vi "Teleop.vi"(10 "Match Info":T1={"Autonomous Elapsed Seconds"=0.0, "TeleOp Elapsed Seconds"=0.0, "Disabled Elapsed Seconds"=0.0, "Visited Autonomous"=FALSE, "Visited TeleOp"=FALSE, "Visited Disabled"=FALSE, "Autonomous Settings"={"Autonomous Style"=enum."Independent", "VI Refnum"=refnum}}, 11 "Call Context":T2) -> ()   [LabVIEW 2015]
doc: "This VI is called for each TeleOp packet received from the DS where the robot is not disabled. It is often used to read from the joysticks and update I/O or to update setpoints for timed control loops. It should complete and return within 20 milliseconds or it may miss DS packets."
uses:
  <vilib>/Rock Robotics/WPI/DriverStation/WPI_DriverStationDerivedRobotMode.ctl
  <vilib>/Rock Robotics/WPI/DriverStation/WPI_DriverStationMatch Info.ctl
  <vilib>/Rock Robotics/Network Tables/NT Read Boolean.vi
  <vilib>/Rock Robotics/Network Tables/NT Read Number.vi
  Team900-VIs/Logitech/F510/F510-X.vi
  <vilib>/Rock Robotics/Network Tables/NT Write Numeric Array.vi
  Robot Global Data.vi
  Team900-VIs/Team900SwerveDrive/Team900SwerveDrive.lvlib
  Team900-VIs/navX Library v2/navX Library v2.lvlib
panel:
  in  "Force Aim":bool=TRUE
  out "Waveform Chart":cluster{dbl, dbl, dbl, dbl}(graph)
  in  "Negate?":bool=TRUE
  in  "Max Wheel Speed (Ticks per tenth of a second?)":dbl=20000.0
  out "Sample Slider 0":dbl(slide) scale=0.0..5.0
  out "Sample Boolean 1":bool
  out "Sample Boolean 0":bool
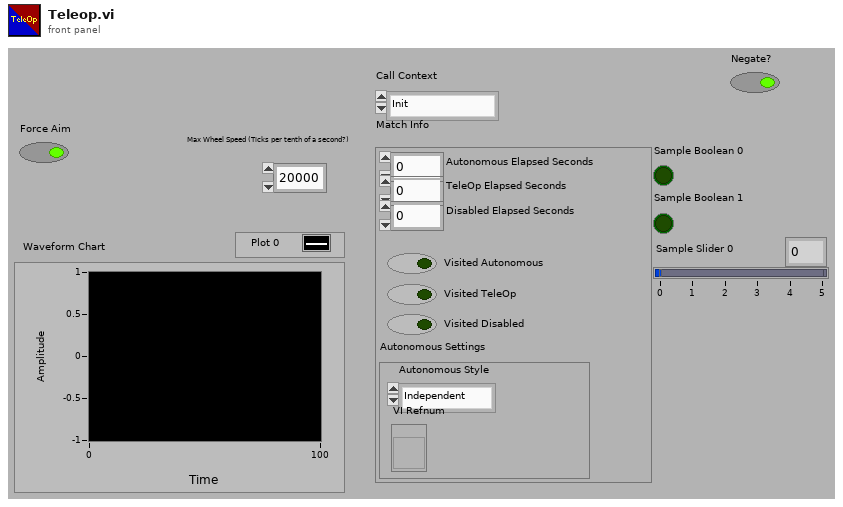
[diagram p1: front panel]
types:
  T1 = typedef "WPI_DriverStationMatch Info.ctl" = cluster{"Autonomous Elapsed Seconds":dbl, "TeleOp Elapsed Seconds":dbl, "Disabled Elapsed Seconds":dbl, "Visited Autonomous":bool, "Visited TeleOp":bool, "Visited Disabled":bool, "Autonomous Settings":cluster{"Autonomous Style":enum16{"Iterative", "Independent"}, "VI Refnum":refnum<vi>}}
  T2 = typedef "WPI_DriverStationDerivedRobotMode.ctl" = enum16{"Init", "Execute", "Stop"}
  T3 = enum16{"nothing", "Fire", "Aim Goal", "Aim Foward"}
  T4 = enum16{"nothing", "intaketotop", "eject ball", "load ball to shooter", "intaketobottom"}
  T5 = cluster{"A":bool, "B":bool, "X":bool, "Y":bool, "LB":bool, "RB":bool, "Back":bool, "Start":bool, "LC":bool, "RC":bool, "LT":bool, "RT":bool}
  T6 = cluster{"Up":bool, "Right":bool, "Down":bool, "Left":bool}
  T7 = typedef "navX Library v2.lvlib/Z900_navX_DeviceTypeDef.ctl" = cluster{"Interface":cluster{"Protocol":T8, "Update Rate (4Hz-60Hz)":u8, "navX Open TypeDef":variant}, "Notify Packet":refnum<notifier>, "Loop VI Refnum":refnum<vi>, "Ready to Close Occurrence Refnum":refnum<k4>}
  T8 = typedef "navX Library v2.lvlib/Z900_navX_ProtocolTypeDef.ctl" = enum16{"SERIAL", "I2C", "SPI"}
  T9 = cluster{"Yaw":dbl, "Roll":dbl, "Pitch":dbl, "Heading":dbl, "Fused Heading":dbl}
  T10 = typedef "WPI_MotorControlDeviceRef.ctl" = cluster{"DeviceStatus":errorcluster, "Type":T11, "PWM":cluster{"PWM Channel":T12, "DeadBand":T13}, "CAN":cluster{"Device Number":u8, "Control Mode":T14, "Semaphore":T15, "Max Vout":dbl, "TalonSRX Control Mode":T16}, "Invert":bool}
  T11 = typedef "WPI_MotorControlType.ctl" = enum16{"PWM", "CAN", "CANTalonSRX"}
  T12 = typedef "FPGA_DIOPWMChannel.ctl" = enum8{"PWM 0", "PWM 1", "PWM 2", "PWM 3", "PWM 4", "PWM 5", "PWM 6", "PWM 7", "PWM 8", "PWM 9", "PWM MXP 0", "PWM MXP 1", "PWM MXP 2", "PWM MXP 3", "PWM MXP 4", "PWM MXP 5", "PWM MXP 6", "PWM MXP 7", "PWM MXP 8", "PWM MXP 9", "Invalid"}
  T13 = typedef "WPI_PWMDeadband.ctl" = cluster{"Name":string, "maxPositivePwm":i32, "minPositivePwm":i32, "centerPwm":i32, "maxNegativePwm":i32, "minNegativePwm":i32, "angularRange":u16}
  T14 = typedef "WPI_CANJaguar_ControlMode.ctl" = enum8{"Percent VBus", "Current", "Speed", "Position", "Voltage"}
  T15 = typedef "Semaphore RefNum" = refnum<k1>
  T16 = typedef "WPI_CANTalonSRX_APIControlMode.ctl" = enum8{"Percent VBus", "Speed", "Position", "Slave", "Unchanged / Invalid", "Voltage Compensation", "Current", "Motion Profile"}
  T17 = typedef "WPI_CANTalonSRX_GlobalStatus.ctl" = cluster{"Applied Throttle":dbl, "Module Enabled":bool, "CAN Error":errorcluster, "Closed Loop Error":dbl, "Forward Limit Switch Closed":bool, "Reverse Limit Switch Closed":bool, "Sensor Position":dbl, "Sensor Velocity":dbl, "Current":dbl, "Sticky Fault - Over Temp":bool, "Sticky Fault - Under Voltage":bool, "Sticky Fault - Forward Limit":bool, "Sticky Fault - Reverse Limit":bool, "Sticky Fault - Forward Soft Limit":bool, "Sticky Fault - Reverse Soft Limit":bool, "Brake is Enabled":bool, "Encoder Position":dbl, "Encoder Velocity":dbl, "Encoder Index Count":dbl, "Encoder A Pin State":bool, "Encoder B Pin State":bool, "Encoder Index Pin State":bool, "Analog In":dbl, "Analog In Velocity":dbl, "Temperature (C)":dbl, "Battery Voltage":dbl, "Control 5 Is Supported":bool, "Current Profile Slot Select":dbl, "Pos Div 8":bool, "Vel Div 4":bool, "Pulse Width Position":i32, "Pulse Width Velocity":i32, "Pulse Width Rise To Rise (us)":i32, "Pulse Width Rise To Fall (us)":i32, "Mot Prof Active Is Under Run":bool, "Mot Prof Active Has Under Run":bool, "Mot Prof Active Is Last":bool, "Mot Prof Active Velocity Only":bool, "Mot Prof Active Is Valid":bool, "Mot Prof Buffer Is Full":bool, "Mot Prof Active Profile Slot Select":i32, "Mot Prof NextID":i32, "Mot Prof Count":i32, "Mot Prof Active Velocity":dbl, "Mot Prof Active Position":dbl, "Mot Prof Output Enable":i32}
  T18 = typedef "WPI_DigitalInputDevRef.ctl" = cluster{"DevStatus":errorcluster, "DIO Channel":T19}
  T19 = typedef "FPGA_DIOChannel.ctl" = enum8{"DIO 0", "DIO 1", "DIO 2", "DIO 3", "DIO 4", "DIO 5", "DIO 6", "DIO 7", "DIO 8", "DIO 9", "DIO MXP 0", "DIO MXP 1", "DIO MXP 2", "DIO MXP 3", "DIO MXP 4", "DIO MXP 5", "DIO MXP 6", "DIO MXP 7", "DIO MXP 8", "DIO MXP 9", "DIO MXP 10", "DIO MXP 11", "DIO MXP 12", "DIO MXP 13", "DIO MXP 14", "DIO MXP 15", "Invalid"}
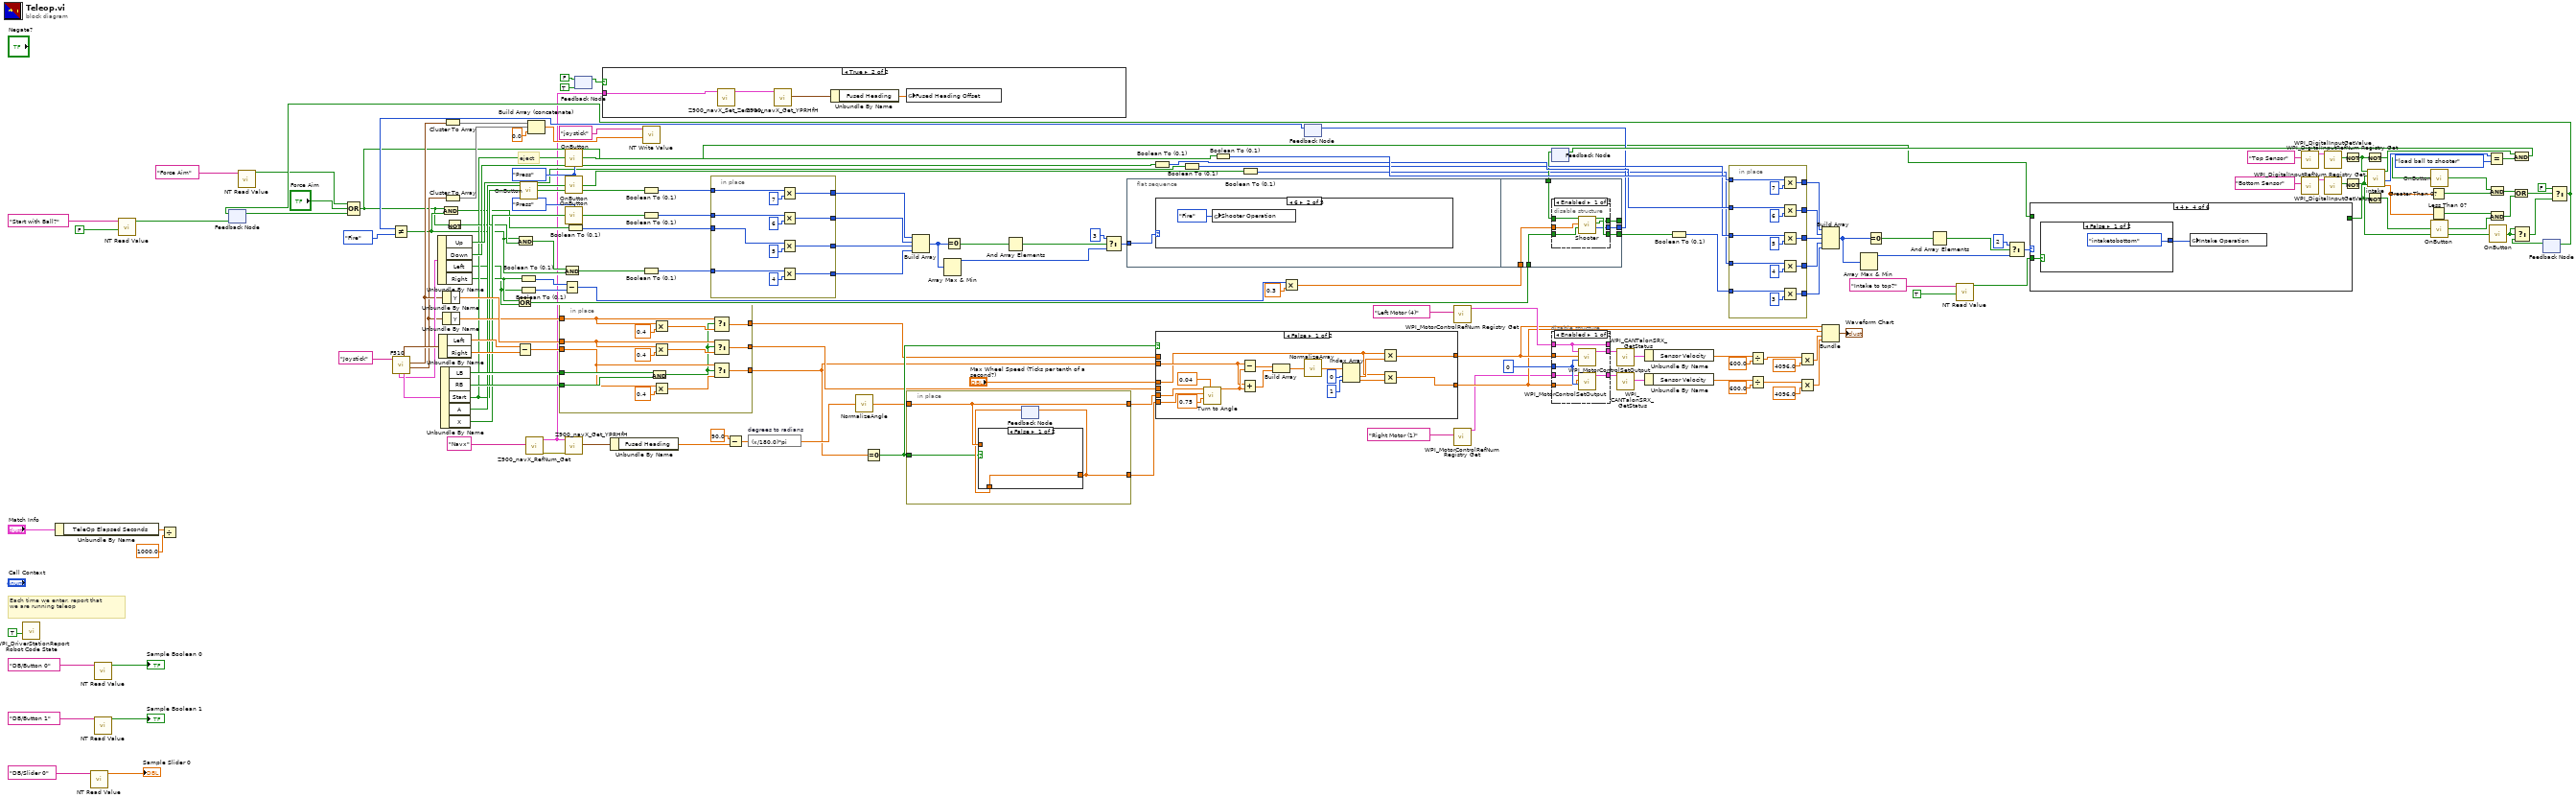
[diagram p0: block diagram]
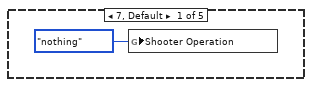
[diagram p4: hidden frame]
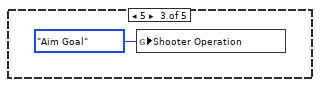
[diagram p5: hidden frame]
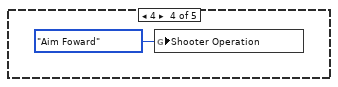
[diagram p6: hidden frame]
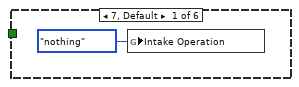
[diagram p9: hidden frame]
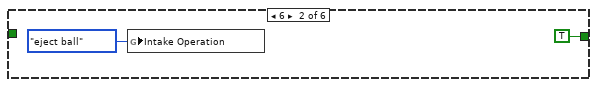
[diagram p10: hidden frame]
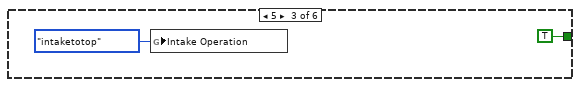
[diagram p11: hidden frame]
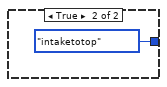
[diagram p12: hidden frame]
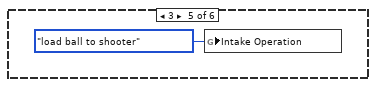
[diagram p13: hidden frame]
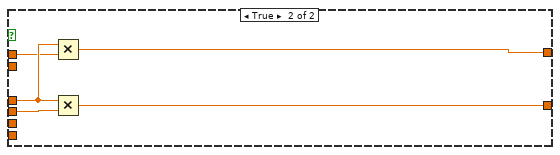
[diagram p16: hidden frame]
diagram:
  w130 = enum16{"Press", "Release", "Both"}."Press" ("Mode")
  # "eject"
  # "Each time we enter, report that\nwe are running teleop"
  n1 = call <vilib>:"WPI_DriverStationReport Robot Code State.vi"("TeleOp"=TRUE ("Autonomous")) -> ()  [unwired: 10 in, 1 out]
  n2 = Unbundle By Name("Match Info") -> ("TeleOp Elapsed Seconds"=w134:dbl)
  n3 = call-poly <vilib>:"NT Read Value.vi"("Name"="DB/Slider 0" ("refnum name")) -> ("Numeric"=→"Sample Slider 0":dbl)  [unwired: 9 in, 1 out]
  n4 = call-poly <vilib>:"NT Read Value.vi"("Name"="DB/Button 0" ("refnum name")) -> ("Boolean"=→"Sample Boolean 0":bool)  [unwired: 9 in, 1 out]
  n5 = call-poly <vilib>:"NT Read Value.vi"("Name"="DB/Button 1" ("refnum name")) -> ("Boolean"=→"Sample Boolean 1":bool)  [unwired: 9 in, 1 out]
  n6 = call-poly <vilib>:"NT Read Value.vi"("Default Value"=FALSE, "Name"="Start with Ball?") -> ("Boolean"=w17:bool)  [unwired: 8 in, 1 out]
  n7 = Divide(x=w134, y=1000.0) -> ()  [unwired: 1 out]
  n8 = feedback #1(w17) -> (w25:bool)
  n9 = call-poly <vilib>:"NT Read Value.vi"("Name"="Force Aim") -> ("Boolean"=w15:bool)  [unwired: 9 in, 1 out]
  n10 = Compound Arithmetic op=OR(w15, "Force Aim", w25) -> (w40:bool)
  n11 = call-poly "F510.vi"("refnum name"="Joystick") -> ("Right Stick"=w74:cluster{"X":dbl, "Y":dbl}, "Left Stick"=w75:cluster{"X":dbl, "Y":dbl}, "Buttons"=w155:T5, "Triggers"=w154:cluster{"Left":dbl, "Right":dbl}, "D-Pad Buttons"=w132:T6)  [unwired: 4 in, 2 out]
  n12 = Unbundle By Name(w132) -> ("Up"=w104:bool, "Down"=w103:bool, "Left"=w6:bool, "Right"=w7:bool)
  n13 = Unbundle By Name(w154) -> ("Left"=w153:dbl, "Right"=w152:dbl)
  n14 = Unbundle By Name(w155) -> ("LB"=w159:bool, "RB"=w160:bool, "Start"=w85:bool, "A"=w131:bool, "X"=w102:bool)
  n15 = Unbundle By Name(w75) -> ("Y"=w157:dbl)
  n16 = Unbundle By Name(w74) -> ("Y"=w158:dbl)
  n17 = Cluster To Array(cluster=w75) -> (array=w73:dbl[])
  n18 = Cluster To Array(cluster=w74) -> (array=w72:dbl[])
  n19 = Not(x=w40) -> (.not. x?=w88:bool)
  n20 = Or(x=w7, y=w6) -> (x .or. y?=w5:bool)
  n21 = Subtract(x=w153, y=w152) -> (x-y=w112:dbl)
  n22 = Boolean To (0,1)(Boolean=w7) -> (0, 1=w12:i16)
  n23 = Boolean To (0,1)(Boolean=w6) -> (0, 1=w11:i16)
  n24 = call "OnButton.vi"("Button"=w85) -> ("Value"=w86:bool)  [unwired: 1 in]
  n25 = call "Z900_navX_RefNum_Get.vi"("refnum name"="Navx") -> ("error out"=w139:errorcluster, "navX Device"=w1:T7)  [unwired: 9 in]
  n26 = Build Array (concatenate)(w73, w72, 0.0) -> (w69:dbl[])
  n27 = in-place {
    in-place-border: w160 -> [w183]
    in-place-border: w159 -> [w182]
    in-place-border: w158 -> [w177]
    in-place-border: w157 -> [w176]
    in-place-border: [w175] -> w79
    in-place-border: [w174] -> w145
    in-place-border: w112 -> [w171]
    in-place-border: [w169] -> w111
    n28 = And(x=w182, y=w183) -> (x .and. y?=w170:bool)
    n29 = Multiply(x=w176, y=0.4) -> (x*y=w179:dbl)
    n30 = Multiply(x=w177, y=0.4) -> (x*y=w181:dbl)
    n31 = Multiply(x=w171, y=0.4) -> (x*y=w173:dbl)
    n32 = Select(t=w176, s=w170, f=w179) -> (s? t:f=w175:dbl)
    n33 = Select(t=w177, s=w170, f=w181) -> (s? t:f=w174:dbl)
    n34 = Select(t=w171, s=w170, f=w173) -> (s? t:f=w169:dbl)
  }
  n35 = Subtract(x=w12, y=w11) -> (x-y=w9:i16)
  n36 = call "OnButton.vi"("Button"=w85, "Mode"=w130) -> ("Value"=w47:bool)
  n37 = call "OnButton.vi"("Button"=w131, "Mode"=w130) -> ("Value"=w43:bool)
  n38 = call "OnButton.vi"("Button"=w102, "Mode"=enum16{"Press", "Release", "Both"}."Press") -> ("Value"=w100:bool)
  n39 = call "Z900_navX_Get_YPRHfH.vi"("error in (no error)"=w139, "navX Device"=w1) -> ("YRPHfH"=w140:T9)  [unwired: 6 in, 3 out]
  n40 = feedback-in #2(FALSE) -> ()
  n41 = feedback #2(TRUE) -> (w3:bool)
  n42 = case shown="True" w3 {
    tunnel: w1 -> [_ w184]
    frame False {
    }
    frame True {
      n43 = call "Z900_navX_Set_ZeroYaw.vi"("navX Device"=w184) -> ("navX Device"=w185:T7)  [unwired: 9 in, 1 out]
      n44 = call "Z900_navX_Get_YPRHfH.vi"("navX Device"=w185) -> ("YRPHfH"=w187:T9)  [unwired: 7 in, 3 out]
      n45 = Unbundle By Name(w187) -> ("Fused Heading"=w186:dbl)
      n46 = global write "Robot Global Data.vi" "Fused Heading Offset"(w186) -> ()
    }
  }
  n47 = Unbundle By Name(w140) -> ("Fused Heading"=w81:dbl)
  n48 = Boolean To (0,1)(Boolean=w86) -> (0, 1=w83:i16)
  n49 = Boolean To (0,1)(Boolean=w100) -> (0, 1=w99:i16)
  n50 = call-poly <vilib>:"NT Write Value.vi"("Numeric Array"=w69, "Name"="joystick") -> ()  [unwired: 9 in, 1 out]
  n51 = Subtract(x=90.0 ("y"), y=w81) -> (x-y=w136:dbl)
  n52 = expression code="(x/180.0)*pi" "degrees to radians"(w136) -> (w143:dbl)
  n53 = call "NormalizeAngle.vi"("angle (rad)"=w143) -> ("angle (between pi and -pi)"=w142:dbl)
  n54 = Equal To 0?(x=w111) -> (x = 0?=w146:bool)
  n55 = in-place {
    in-place-border: w142 -> [w191]
    in-place-border: w146 -> [w188]
    in-place-border: [w191] -> w144
    in-place-border: [w189] -> w141
    n56 = feedback #3() -> (w190:dbl)  [unwired: 1 in]
    n57 = case shown="False" w188 {
      tunnel: w191 -> [_ w193]
      tunnel: [w192 w193] -> w189
      tunnel: w190 -> [w192 _]
      frame False {
      }
      frame True {
      }
    }
    n58 = feedback-in #3(w189) -> ()
  }
  n59 = flat-sequence {
    tunnel: w87 -> [w194]
    tunnel: w82 -> [w204]
    tunnel: [w203] -> _
    tunnel: [w202] -> w48
    tunnel: [w201] -> w80
    tunnel: w8 -> [w200]
    tunnel: w5 -> [w199]
    frame #0 {
      n60 = case shown="6" w194 {
        frame 7, Default {
          n61 = global write "Robot Global Data.vi" "Shooter Operation"(T3."nothing" ("Shooter Operation")) -> ()
        }
        frame 6 {
          n62 = global write "Robot Global Data.vi" "Shooter Operation"(T3."Fire" ("y")) -> ()
        }
        frame 5 {
          n63 = global write "Robot Global Data.vi" "Shooter Operation"(T3."Aim Goal" ("Shooter Operation")) -> ()
        }
        frame 4 {
          n64 = global write "Robot Global Data.vi" "Shooter Operation"(T3."Aim Foward" ("Shooter Operation")) -> ()
        }
        frame 3 {
        }
      }
    }
    frame #1 {
      n65 = disable-structure shown="Enabled" {
        disable-tunnel: [w210 _] -> w202
        disable-tunnel: w204 -> [w209 _]
        disable-tunnel: [w208 _] -> w201
        disable-tunnel: [w207 _] -> w203
        disable-tunnel: w200 -> [w206 _]
        disable-tunnel: w199 -> [w205 _]
        frame Enabled {
          n66 = call "Shooter.vi"("Override?"=w205, "Override Setpoint"=w206, "Load Ball Finished"=w209) -> ("Shooter Operation"=w208:T3, "Finished"=w207:bool, "Load Ball"=w210:bool)  [unwired: 5 in, 1 out]
        }
        frame Disabled {
        }
      }
    }
  }
  n67 = Boolean To (0,1)(Boolean=w103) -> (0, 1=w128:i16)
  n68 = case shown="False" w146 {
    tunnel: "Max Wheel Speed (Ticks per tenth of a second?)" -> [w213 w230]
    tunnel: [w225 w231] -> w67
    tunnel: [w226 w232] -> w68
    tunnel: w144 -> [w211 _]
    tunnel: w111 -> [w222 _]
    tunnel: w79 -> [_ w229]
    tunnel: w145 -> [_ w228]
    tunnel: w141 -> [w212 _]
    frame False {
      n69 = call "Turn to Angle.vi"("Angle Tolerance"=0.04, "Rotation Multiplier"=0.75, "Target angle"=w212, "Angle (radians; 0 = right)"=w211) -> ("Turn Set Point"=w223:dbl)  [unwired: 3 in, 1 out]
      n70 = Subtract(x=w222, y=w223) -> (x-y=w221:dbl)
      n71 = Add(x=w222, y=w223) -> (x+y=w214:dbl)
      n72 = Build Array(w221, w214) -> (w220:dbl[])
      n73 = call "NormalizeArray.vi"("array"=w220) -> ("normalized array"=w219:dbl[])
      n74 = Index Array(array=w219, index #1=0 ("index"), index #2=1 ("index")) -> (element #1=w216:dbl, element #2=w215:dbl)
      n75 = Multiply(x=w213, y=w216) -> (x*y=w226:dbl)
      n76 = Multiply(x=w213, y=w215) -> (x*y=w225:dbl)
    }
    frame True {
      n77 = Multiply(x=w230, y=w229) -> (x*y=w232:dbl)
      n78 = Multiply(x=w230, y=w228) -> (x*y=w231:dbl)
    }
  }
  n79 = Boolean To (0,1)(Boolean=w104) -> (0, 1=w127:i16)
  n80 = Boolean To (0,1)(Boolean=w47) -> (0, 1=w129:i16)
  n81 = Boolean To (0,1)(Boolean=w43) -> (0, 1=w46:i16)
  n82 = Multiply(x=w9, y=0.3) -> (x*y=w8:dbl)
  n83 = feedback #4() -> (w77:T3)  [unwired: 1 in]
  n84 = Not Equal?(x=w77, y=T3."Fire") -> (x != y?=w49:bool)
  n85 = And(x=w40, y=w49) -> (x .and. y?=w41:bool)
  n86 = And(x=w49, y=w88) -> (x .and. y?=w50:bool)
  n87 = And(x=w50, y=w49) -> (x .and. y?=w78:bool)
  n88 = Boolean To (0,1)(Boolean=w41) -> (0, 1=w90:i16)
  n89 = Boolean To (0,1)(Boolean=w78) -> (0, 1=w89:i16)
  n90 = in-place {
    in-place-border: w99 -> [w244]
    in-place-border: w90 -> [w241]
    in-place-border: w89 -> [w239]
    in-place-border: [w238] -> w93
    in-place-border: [w237] -> w92
    in-place-border: [w236] -> w91
    in-place-border: w83 -> [w234]
    in-place-border: [w233] -> w84
    n91 = Multiply(x=w234, y=i16 7) -> (x*y=w233:i16)
    n92 = Multiply(x=w244, y=i16 6) -> (x*y=w238:i16)
    n93 = Multiply(x=w241, y=i16 5) -> (x*y=w237:i16)
    n94 = Multiply(x=w239, y=i16 4) -> (x*y=w236:i16)
  }
  n95 = Build Array(w84, w93, w92, w91) -> (w98:i16[])
  n96 = Array Max & Min(array=w98) -> (max value=w94:i16)  [unwired: 3 out]
  n97 = Equal To 0?(x=w98) -> (x = 0?=w97:bool[])
  n98 = And Array Elements(Boolean array=w97) -> (logical AND=w96:bool)
  n99 = Select(t=3, s=w96, f=w94) -> (s? t:f=w87:i32)
  n100 = feedback-in #4(w80) -> ()
  n101 = call <vilib>:"WPI_MotorControlRefNum Registry Get.vi"("refnum name"="Left Motor (4)") -> ("MotorControlDevRef"=w148:T10)  [unwired: 9 in, 1 out]
  n102 = call <vilib>:"WPI_MotorControlRefNum Registry Get.vi"("refnum name"="Right Motor (1)") -> ("MotorControlDevRef"=w66:T10)  [unwired: 9 in, 1 out]
  n103 = feedback #5() -> (w82:bool)  [unwired: 1 in]
  n104 = disable-structure shown="Enabled" {
    disable-tunnel: u8 0 ("Sync Group / Parameter Slot") -> [w251 _]
    disable-tunnel: w66 -> [w250 _]
    disable-tunnel: w148 -> [w247 _]
    disable-tunnel: w68 -> [w249 _]
    disable-tunnel: w67 -> [w248 _]
    disable-tunnel: [w247 _] -> _
    disable-tunnel: [w246 _] -> w65
    disable-tunnel: [w245 _] -> w64
    frame Enabled {
      n105 = call <vilib>:"WPI_MotorControlSetOutput.vi"("Sync Group / Parameter Slot"=w251, "Output"=w249, "MotorControlDevRef"=w247) -> ("MotorControlDevRef"=w246:T10)  [unwired: 6 in, 2 out]
      n106 = call <vilib>:"WPI_MotorControlSetOutput.vi"("Sync Group / Parameter Slot"=w251, "Output"=w248, "MotorControlDevRef"=w250) -> ("MotorControlDevRef"=w245:T10)  [unwired: 6 in, 2 out]
    }
    frame Disabled {
    }
  }
  n107 = call <vilib>:"WPI_CANTalonSRX_GetStatus.vi"("CAN Talon SRX Ref"=w65) -> ("Talon SRX Status"=w62:T17)  [unwired: 8 in, 2 out]
  n108 = call <vilib>:"WPI_CANTalonSRX_GetStatus.vi"("CAN Talon SRX Ref"=w64) -> ("Talon SRX Status"=w63:T17)  [unwired: 8 in, 2 out]
  n109 = Unbundle By Name(w62) -> ("Sensor Velocity"=w61:dbl)
  n110 = Unbundle By Name(w63) -> ("Sensor Velocity"=w54:dbl)
  n111 = Boolean To (0,1)(Boolean=w48) -> (0, 1=w126:i16)
  n112 = in-place {
    in-place-border: w129 -> [w266]
    in-place-border: w128 -> [w263]
    in-place-border: w127 -> [w261]
    in-place-border: w126 -> [w260]
    in-place-border: [w258] -> w125
    in-place-border: [w257] -> w124
    in-place-border: [w256] -> w123
    in-place-border: [w255] -> w44
    in-place-border: w46 -> [w253]
    in-place-border: [w252] -> w45
    n113 = Multiply(x=w266, y=i16 7) -> (x*y=w258:i16)
    n114 = Multiply(x=w263, y=i16 6) -> (x*y=w257:i16)
    n115 = Multiply(x=w261, y=i16 5) -> (x*y=w256:i16)
    n116 = Multiply(x=w253, y=i16 4) -> (x*y=w252:i16)
    n117 = Multiply(x=w260, y=i16 3) -> (x*y=w255:i16)
  }
  n118 = Divide(x=w61, y=600.0) -> (x/y=w59:dbl)
  n119 = Divide(x=w54, y=600.0) -> (x/y=w55:dbl)
  n120 = Multiply(x=w59, y=4096.0) -> (x*y=w52:dbl)
  n121 = Multiply(x=w55, y=4096.0) -> (x*y=w53:dbl)
  n122 = Build Array(w125, w124, w123, w45, w44) -> (w110:i16[])
  n123 = Bundle(w68, w67, w52, w53) -> (→"Waveform Chart":cluster{dbl, dbl, dbl, dbl})  [unwired: 1 in]
  n124 = Array Max & Min(array=w110) -> (max value=w105:i16)  [unwired: 3 out]
  n125 = Equal To 0?(x=w110) -> (x = 0?=w109:bool[])
  n126 = And Array Elements(Boolean array=w109) -> (logical AND=w108:bool)
  n127 = call-poly <vilib>:"NT Read Value.vi"("Default Value"=TRUE, "Name"="Intake to top?") -> ("Boolean"=w113:bool)  [unwired: 8 in, 1 out]
  n128 = Select(t=2, s=w108, f=w105) -> (s? t:f=w106:i32)
  n129 = case shown="4" w106 {
    tunnel: [_ TRUE TRUE _ _ _] -> w122
    tunnel: w113 -> [_ _ _ w272 _ _]
    tunnel: w40 -> [_ _ _ _ _ _]
    frame 7, Default {
      n130 = global write "Robot Global Data.vi" "Intake Operation"(T4."nothing" ("Intake Operation")) -> ()
    }
    frame 6 {
      n131 = global write "Robot Global Data.vi" "Intake Operation"(T4."eject ball" ("Intake Operation")) -> ()
    }
    frame 5 {
      n132 = global write "Robot Global Data.vi" "Intake Operation"(T4."intaketotop" ("Intake Operation")) -> ()
    }
    frame 4 {
      n133 = case shown="False" w272 {
        tunnel: [T4."intaketobottom" ("Intake Operation") T4."intaketotop" ("Intake Operation")] -> w273
        frame False {
        }
        frame True {
        }
      }
      n134 = global write "Robot Global Data.vi" "Intake Operation"(w273) -> ()
    }
    frame 3 {
      n135 = global write "Robot Global Data.vi" "Intake Operation"(T4."load ball to shooter" ("Intake Operation")) -> ()
    }
    frame 2 {
    }
  }
  n136 = call <vilib>:"WPI_DigitalInputRefNum Registry Get.vi"("refnum name"="Top Sensor") -> ("DigitalInputDevRef"=w135:T18)  [unwired: 9 in, 1 out]
  n137 = call <vilib>:"WPI_DigitalInputRefNum Registry Get.vi"("refnum name"="Bottom Sensor") -> ("DigitalInputDevRef"=w30:T18)  [unwired: 9 in, 1 out]
  n138 = call <vilib>:"WPI_DigitalInputGetValue.vi"("DigitalInputDevRef"=w135) -> ("Value"=w114:bool)  [unwired: 8 in, 2 out]
  n139 = call <vilib>:"WPI_DigitalInputGetValue.vi"("DigitalInputDevRef"=w30) -> ("Value"=w29:bool)  [unwired: 8 in, 2 out]
  n140 = Not(x=w114) -> (.not. x?=w36:bool)
  n141 = Not(x=w29) -> (.not. x?=w34:bool)
  n142 = Not(x=w36) -> (.not. x?=w35:bool)
  n143 = Not(x=w34) -> (.not. x?=w23:bool)
  n144 = call "intake.vi"("Manuel Mode"=w122, "Bottom Sensor"=w34, "Top Sensor"=w36) -> ("Elevater VBUS"=w21:dbl, "Intake Operation"=w119:T4, "Operation finished"=w116:bool)  [unwired: 5 in, 1 out]
  n145 = Greater Than 0?(x=w21) -> (x > 0?=w14:bool)
  n146 = Less Than 0?(x=w21) -> (x < 0?=w13:bool)
  n147 = call "OnButton.vi"("Button"=w35) -> ("Value"=w24:bool)  [unwired: 1 in]
  n148 = call "OnButton.vi"("Button"=w23) -> ("Value"=w33:bool)  [unwired: 1 in]
  n149 = Equal?(x=w119, y=T4."load ball to shooter") -> (x = y?=w117:bool)
  n150 = And(x=w24, y=w14) -> (x .and. y?=w20:bool)
  n151 = And(x=w13, y=w33) -> (x .and. y?=w22:bool)
  n152 = call "OnButton.vi"("Button"=w34) -> ("Value"=w38:bool)  [unwired: 1 in]
  n153 = Or(x=w20, y=w22) -> (x .or. y?=w27:bool)
  n154 = And(x=w116, y=w117) -> (x .and. y?=w115:bool)
  n155 = feedback-in #5(w115) -> ()
  n156 = feedback #6() -> (w37:bool)  [unwired: 1 in]
  n157 = Select(t=w38, s=w38, f=w37) -> (s? t:f=w32:bool)
  n158 = Select(t=FALSE, s=w27, f=w32) -> (s? t:f=w26:bool)
  n159 = feedback-in #1(w26) -> ()
  n160 = feedback-in #6(w26) -> ()
